vi "Little-Endian Bytes To Words I32.vi"(1 "bytes in":u8[](array[numeric]) format="%02x") -> (0 "words out":i32[](array[numeric]))   [LabVIEW 2020, in "NI_Bit Manipulation.lvlib"]
uses:
  <vilib>/Bit Manipulation/NI_Bit Manipulation.lvlib
  068ac748-d2cd-4c9a-8044-fc563640b5b0.vi
  068ac748-d2cd-4c9a-8044-fc563640b5b0.vi/9c6d32c5-bf1b-4c5c-8cfa-b02aa5dc3cd4.vi
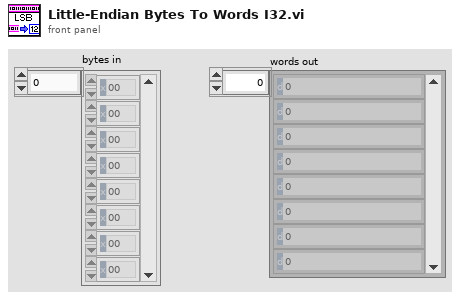
[diagram p1: front panel]
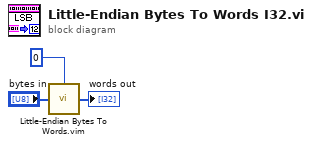
[diagram p0: block diagram]
diagram:
  n1 = call "Little-Endian Bytes To Words.vim"("bytes in"="bytes in", "word type"=0) -> ("words out"=→"words out":i32[])
